vi "Lab Panel V5.22.1.vi"() -> ()   [LabVIEW 2013] (continued)
            n2200 = Equal?(x=w3894, y=w3895) -> (x = y?=w3879:bool)
            n2201 = stacked-sequence {
              tunnel: w3893 -> [w3903 _ _ _ _ _ _ _ _ _]
              tunnel: w3892 -> [_ w3979 _ _ _ _ _ _ _ _]
              tunnel: w3891 -> [_ _ w4059 _ _ _ _ _ _ _]
              tunnel: w3890 -> [_ _ _ w4139 _ _ _ _ _ _]
              tunnel: w3889 -> [_ _ _ _ w4219 _ _ _ _ _]
              tunnel: w3888 -> [_ _ _ _ _ w4299 _ _ _ _]
              tunnel: w3887 -> [_ _ _ _ _ _ w4379 _ _ _]
              tunnel: w3886 -> [_ _ _ _ _ _ _ w4459 _ _]
              tunnel: w3885 -> [_ _ _ _ _ _ _ _ w4539 _]
              tunnel: w3884 -> [_ _ _ _ _ _ _ _ _ w4619]
              tunnel: w3881 -> [w3902 w3983 w4063 w4143 w4223 w4303 w4383 w4463 w4543 w4623]
              tunnel: w3880 -> [w3901 w3982 w4062 w4142 w4222 w4302 w4382 w4462 w4542 w4622]
              tunnel: w3879 -> [w3900 w3981 w4061 w4141 w4221 w4301 w4381 w4461 w4541 w4621]
              tunnel: w3878 -> [w3899 w3980 w4060 w4140 w4220 w4300 w4380 w4460 w4540 w4620]
              frame #0 {
                n2202 = case shown="True" w3903 {
                  tunnel: w3902 -> [_ w3908]
                  tunnel: w3901 -> [_ w3907]
                  tunnel: w3900 -> [_ w3905]
                  tunnel: w3899 -> [_ w3904]
                  frame False {
                  }
                  frame True {
                    n2203 = local read "DISP LAB01-1"() -> (w3909:T4)
                    n2204 = local read "SIG LAB01-1"() -> (w3910:T2)
                    n2205 = local read "ON L01-1"() -> (w3906:cluster{"amps":dbl, "volts":dbl, "pf":dbl})
                    n2206 = Unbundle(w3910) -> ("AMPS"=w3916:dbl, "VOLTS"=w3914:dbl, "PF"=w3913:dbl, "Tmp Live"=w3912:dbl, "Tmp Neut"=w3915:dbl)
                    n2207 = Unbundle(w3909) -> ("CYCLE"=w3911:dbl)  [unwired: 2 out]
                    n2208 = stacked-sequence {
                      tunnel: w3916 -> [w3920 w3939]
                      tunnel: w3915 -> [_ w3938]
                      tunnel: w3914 -> [w3919 w3937]
                      tunnel: w3913 -> [w3918 w3936]
                      tunnel: w3912 -> [_ w3935]
                      tunnel: w3911 -> [_ w3934]
                      tunnel: w3908 -> [_ w3933]
                      tunnel: w3907 -> [w3921 _]
                      tunnel: w3906 -> [w3917 w3931]
                      tunnel: w3905 -> [_ w3932]
                      tunnel: w3904 -> [_ w3927]
                      frame #0 {
                        n2209 = case shown="True" w3921 {
                          tunnel: w3920 -> [_ w3926]
                          tunnel: w3919 -> [_ w3925]
                          tunnel: w3918 -> [_ w3924]
                          tunnel: w3917 -> [_ w3922]
                          frame False {
                          }
                          frame True {
                            n2210 = Bundle(cluster=w3922, "amps"=w3926, "volts"=w3925, "pf"=w3924) -> (w3923:cluster{"amps":dbl, "volts":dbl, "pf":dbl})
                            n2211 = local write "ON L01-1"(w3923) -> ()
                          }
                        }
                      }
                      frame #1 {
                        n2212 = Unbundle(w3931) -> ("amps"=w3930:dbl, "volts"=w3929:dbl, "pf"=w3928:dbl)
                        n2213 = case shown="True" w3932 {
                          tunnel: w3939 -> [_ w3940]
                          tunnel: w3938 -> [_ w3978]
                          tunnel: w3937 -> [_ _]
                          tunnel: w3936 -> [_ _]
                          tunnel: w3935 -> [_ w3977]
                          tunnel: w3934 -> [_ w3976]
                          tunnel: w3933 -> [_ w3944]
                          tunnel: w3930 -> [_ w3941]
                          tunnel: w3929 -> [_ w3973]
                          tunnel: w3928 -> [_ w3972]
                          tunnel: w3927 -> [_ w3942]
                          frame False {
                          }
                          frame True {
                            n2214 = local read "TDMS LAB01-1"() -> (w3975:refnum<k34>)
                            n2215 = Build Array(w3973) -> (w3969:dbl[])
                            n2216 = Build Array(w3972) -> (w3968:dbl[])
                            n2217 = Build Array(w3977) -> (w3967:dbl[])
                            n2218 = Build Array(w3978) -> (w3966:dbl[])
                            n2219 = Build Array(w3941) -> (w3971:dbl[])
                            n2220 = Build Array(w3940) -> (w3970:dbl[])
                            n2221 = Build Array(w3976) -> (w3965:dbl[])
                            n2222 = Build Array("AMPS ON", "AMPS OFF", "VOLTS", "PF", "TEMP Live", "TEMP Neut", "CYCLE") -> (w3949:string[])
                            n2223 = Bundle By Name("Y"=w3971, "t0"=w3942) -> (w3964:waveform(dbl))  [unwired: 1 in]
                            n2224 = Bundle By Name("Y"=w3970, "t0"=w3942) -> (w3963:waveform(dbl))  [unwired: 1 in]
                            n2225 = Bundle By Name("Y"=w3969, "t0"=w3942) -> (w3962:waveform(dbl))  [unwired: 1 in]
                            n2226 = Bundle By Name("Y"=w3968, "t0"=w3942) -> (w3961:waveform(dbl))  [unwired: 1 in]
                            n2227 = Bundle By Name("Y"=w3967, "t0"=w3942) -> (w3960:waveform(dbl))  [unwired: 1 in]
                            n2228 = Bundle By Name("Y"=w3966, "t0"=w3942) -> (w3959:waveform(dbl))  [unwired: 1 in]
                            n2229 = Bundle By Name("Y"=w3965, "t0"=w3942) -> (w3958:waveform(dbl))  [unwired: 1 in]
                            n2230 = Build Array(w3964, w3963, w3962, w3961, w3960, w3959, w3958) -> (w3957:waveform(dbl)[])
                            n2231 = TDMS Write(0:w3975, 5:"TEST VALUES", 7:w3949, 9:w3957) -> (4:w3948:refnum<k34>, 6:w3947:string, 15:w3946:errorcluster)  [unwired: 2 in, 1 out]
                            n2232 = TDMS Write(0:w3948, 5:w3947, 7:"TIME", 9:w3944, 11:w3946) -> (15:w3943:errorcluster)  [unwired: 1 in, 3 out]
                            n2233 = local write "data file error"(w3943) -> ()
                          }
                        }
                      }
                    }
                  }
                }
              }
              frame #1 {
                n2234 = case shown="True" w3979 {
                  tunnel: w3983 -> [_ w3988]
                  tunnel: w3982 -> [_ w3987]
                  tunnel: w3981 -> [_ w3985]
                  tunnel: w3980 -> [_ w3984]
                  frame False {
                  }
                  frame True {
                    n2235 = local read "DISP LAB01-2"() -> (w3989:T4)
                    n2236 = local read "SIG LAB01-2"() -> (w3990:T2)
                    n2237 = local read "ON L01-2"() -> (w3986:cluster{"amps":dbl, "volts":dbl, "pf":dbl})
                    n2238 = Unbundle(w3990) -> ("AMPS"=w3996:dbl, "VOLTS"=w3994:dbl, "PF"=w3993:dbl, "Tmp Live"=w3992:dbl, "Tmp Neut"=w3995:dbl)
                    n2239 = Unbundle(w3989) -> ("CYCLE"=w3991:dbl)  [unwired: 2 out]
                    n2240 = stacked-sequence {
                      tunnel: w3996 -> [w4000 w4019]
                      tunnel: w3995 -> [_ w4018]
                      tunnel: w3994 -> [w3999 w4017]
                      tunnel: w3993 -> [w3998 w4016]
                      tunnel: w3992 -> [_ w4015]
                      tunnel: w3991 -> [_ w4014]
                      tunnel: w3988 -> [_ w4013]
                      tunnel: w3987 -> [w4001 _]
                      tunnel: w3986 -> [w3997 w4011]
                      tunnel: w3985 -> [_ w4012]
                      tunnel: w3984 -> [_ w4007]
                      frame #0 {
                        n2241 = case shown="True" w4001 {
                          tunnel: w4000 -> [_ w4006]
                          tunnel: w3999 -> [_ w4005]
                          tunnel: w3998 -> [_ w4004]
                          tunnel: w3997 -> [_ w4002]
                          frame False {
                          }
                          frame True {
                            n2242 = Bundle(cluster=w4002, "amps"=w4006, "volts"=w4005, "pf"=w4004) -> (w4003:cluster{"amps":dbl, "volts":dbl, "pf":dbl})
                            n2243 = local write "ON L01-2"(w4003) -> ()
                          }
                        }
                      }
                      frame #1 {
                        n2244 = Unbundle(w4011) -> ("amps"=w4010:dbl, "volts"=w4009:dbl, "pf"=w4008:dbl)
                        n2245 = case shown="True" w4012 {
                          tunnel: w4019 -> [_ w4051]
                          tunnel: w4018 -> [_ w4058]
                          tunnel: w4017 -> [_ _]
                          tunnel: w4016 -> [_ _]
                          tunnel: w4015 -> [_ w4057]
                          tunnel: w4014 -> [_ w4056]
                          tunnel: w4013 -> [_ w4021]
                          tunnel: w4010 -> [_ w4053]
                          tunnel: w4009 -> [_ w4052]
                          tunnel: w4008 -> [_ w4050]
                          tunnel: w4007 -> [_ w4042]
                          frame False {
                          }
                          frame True {
                            n2246 = local read "TDMS LAB01-2"() -> (w4055:refnum<k34>)
                            n2247 = Build Array(w4052) -> (w4047:dbl[])
                            n2248 = Build Array(w4050) -> (w4046:dbl[])
                            n2249 = Build Array(w4057) -> (w4045:dbl[])
                            n2250 = Build Array(w4058) -> (w4044:dbl[])
                            n2251 = Build Array(w4053) -> (w4049:dbl[])
                            n2252 = Build Array(w4051) -> (w4048:dbl[])
                            n2253 = Build Array(w4056) -> (w4043:dbl[])
                            n2254 = Build Array("AMPS ON", "AMPS OFF", "VOLTS", "PF", "TEMP Live", "TEMP Neut", "CYCLE") -> (w4026:string[])
                            n2255 = Bundle By Name("Y"=w4049, "t0"=w4042) -> (w4041:waveform(dbl))  [unwired: 1 in]
                            n2256 = Bundle By Name("Y"=w4048, "t0"=w4042) -> (w4040:waveform(dbl))  [unwired: 1 in]
                            n2257 = Bundle By Name("Y"=w4047, "t0"=w4042) -> (w4039:waveform(dbl))  [unwired: 1 in]
                            n2258 = Bundle By Name("Y"=w4046, "t0"=w4042) -> (w4038:waveform(dbl))  [unwired: 1 in]
                            n2259 = Bundle By Name("Y"=w4045, "t0"=w4042) -> (w4037:waveform(dbl))  [unwired: 1 in]
                            n2260 = Bundle By Name("Y"=w4044, "t0"=w4042) -> (w4036:waveform(dbl))  [unwired: 1 in]
                            n2261 = Bundle By Name("Y"=w4043, "t0"=w4042) -> (w4035:waveform(dbl))  [unwired: 1 in]
                            n2262 = Build Array(w4041, w4040, w4039, w4038, w4037, w4036, w4035) -> (w4034:waveform(dbl)[])
                            n2263 = TDMS Write(0:w4055, 5:"TEST VALUES", 7:w4026, 9:w4034) -> (4:w4025:refnum<k34>, 6:w4024:string, 15:w4023:errorcluster)  [unwired: 2 in, 1 out]
                            n2264 = TDMS Write(0:w4025, 5:w4024, 7:"TIME", 9:w4021, 11:w4023) -> (15:w4020:errorcluster)  [unwired: 1 in, 3 out]
                            n2265 = local write "data file error"(w4020) -> ()
                          }
                        }
                      }
                    }
                  }
                }
              }
              frame #2 {
                n2266 = case shown="True" w4059 {
                  tunnel: w4063 -> [_ w4068]
                  tunnel: w4062 -> [_ w4067]
                  tunnel: w4061 -> [_ w4065]
                  tunnel: w4060 -> [_ w4064]
                  frame False {
                  }
                  frame True {
                    n2267 = local read "DISP LAB02-1"() -> (w4069:T4)
                    n2268 = local read "SIG LAB02-1"() -> (w4070:T2)
                    n2269 = local read "ON L02-1"() -> (w4066:cluster{"amps":dbl, "volts":dbl, "pf":dbl})
                    n2270 = Unbundle(w4070) -> ("AMPS"=w4076:dbl, "VOLTS"=w4074:dbl, "PF"=w4073:dbl, "Tmp Live"=w4072:dbl, "Tmp Neut"=w4075:dbl)
                    n2271 = Unbundle(w4069) -> ("CYCLE"=w4071:dbl)  [unwired: 2 out]
                    n2272 = stacked-sequence {
                      tunnel: w4076 -> [w4080 w4099]
                      tunnel: w4075 -> [_ w4098]
                      tunnel: w4074 -> [w4079 w4097]
                      tunnel: w4073 -> [w4078 w4096]
                      tunnel: w4072 -> [_ w4095]
                      tunnel: w4071 -> [_ w4094]
                      tunnel: w4068 -> [_ w4093]
                      tunnel: w4067 -> [w4081 _]
                      tunnel: w4066 -> [w4077 w4091]
                      tunnel: w4065 -> [_ w4092]
                      tunnel: w4064 -> [_ w4087]
                      frame #0 {
                        n2273 = case shown="True" w4081 {
                          tunnel: w4080 -> [_ w4086]
                          tunnel: w4079 -> [_ w4085]
                          tunnel: w4078 -> [_ w4084]
                          tunnel: w4077 -> [_ w4082]
                          frame False {
                          }
                          frame True {
                            n2274 = Bundle(cluster=w4082, "amps"=w4086, "volts"=w4085, "pf"=w4084) -> (w4083:cluster{"amps":dbl, "volts":dbl, "pf":dbl})
                            n2275 = local write "ON L02-1"(w4083) -> ()
                          }
                        }
                      }
                      frame #1 {
                        n2276 = Unbundle(w4091) -> ("amps"=w4090:dbl, "volts"=w4089:dbl, "pf"=w4088:dbl)
                        n2277 = case shown="True" w4092 {
                          tunnel: w4099 -> [_ w4131]
                          tunnel: w4098 -> [_ w4138]
                          tunnel: w4097 -> [_ _]
                          tunnel: w4096 -> [_ _]
                          tunnel: w4095 -> [_ w4137]
                          tunnel: w4094 -> [_ w4136]
                          tunnel: w4093 -> [_ w4101]
                          tunnel: w4090 -> [_ w4133]
                          tunnel: w4089 -> [_ w4132]
                          tunnel: w4088 -> [_ w4130]
                          tunnel: w4087 -> [_ w4122]
                          frame False {
                          }
                          frame True {
                            n2278 = local read "TDMS LAB02-1"() -> (w4135:refnum<k34>)
                            n2279 = Build Array(w4132) -> (w4127:dbl[])
                            n2280 = Build Array(w4130) -> (w4126:dbl[])
                            n2281 = Build Array(w4137) -> (w4125:dbl[])
                            n2282 = Build Array(w4138) -> (w4124:dbl[])
                            n2283 = Build Array(w4133) -> (w4129:dbl[])
                            n2284 = Build Array(w4131) -> (w4128:dbl[])
                            n2285 = Build Array(w4136) -> (w4123:dbl[])
                            n2286 = Build Array("AMPS ON", "AMPS OFF", "VOLTS", "PF", "TEMP Live", "TEMP Neut", "CYCLE") -> (w4106:string[])
                            n2287 = Bundle By Name("Y"=w4129, "t0"=w4122) -> (w4121:waveform(dbl))  [unwired: 1 in]
                            n2288 = Bundle By Name("Y"=w4128, "t0"=w4122) -> (w4120:waveform(dbl))  [unwired: 1 in]
                            n2289 = Bundle By Name("Y"=w4127, "t0"=w4122) -> (w4119:waveform(dbl))  [unwired: 1 in]
                            n2290 = Bundle By Name("Y"=w4126, "t0"=w4122) -> (w4118:waveform(dbl))  [unwired: 1 in]
                            n2291 = Bundle By Name("Y"=w4125, "t0"=w4122) -> (w4117:waveform(dbl))  [unwired: 1 in]
                            n2292 = Bundle By Name("Y"=w4124, "t0"=w4122) -> (w4116:waveform(dbl))  [unwired: 1 in]
                            n2293 = Bundle By Name("Y"=w4123, "t0"=w4122) -> (w4115:waveform(dbl))  [unwired: 1 in]
                            n2294 = Build Array(w4121, w4120, w4119, w4118, w4117, w4116, w4115) -> (w4114:waveform(dbl)[])
                            n2295 = TDMS Write(0:w4135, 5:"TEST VALUES", 7:w4106, 9:w4114) -> (4:w4105:refnum<k34>, 6:w4104:string, 15:w4103:errorcluster)  [unwired: 2 in, 1 out]
                            n2296 = TDMS Write(0:w4105, 5:w4104, 7:"TIME", 9:w4101, 11:w4103) -> (15:w4100:errorcluster)  [unwired: 1 in, 3 out]
                            n2297 = local write "data file error"(w4100) -> ()
                          }
                        }
                      }
                    }
                  }
                }
              }
              frame #3 {
                n2298 = case shown="True" w4139 {
                  tunnel: w4143 -> [_ w4148]
                  tunnel: w4142 -> [_ w4147]
                  tunnel: w4141 -> [_ w4145]
                  tunnel: w4140 -> [_ w4144]
                  frame False {
                  }
                  frame True {
                    n2299 = local read "DISP LAB02-2"() -> (w4149:T4)
                    n2300 = local read "SIG LAB02-2"() -> (w4150:T2)
                    n2301 = local read "ON L02-2"() -> (w4146:cluster{"amps":dbl, "volts":dbl, "pf":dbl})
                    n2302 = Unbundle(w4150) -> ("AMPS"=w4156:dbl, "VOLTS"=w4154:dbl, "PF"=w4153:dbl, "Tmp Live"=w4152:dbl, "Tmp Neut"=w4155:dbl)
                    n2303 = Unbundle(w4149) -> ("CYCLE"=w4151:dbl)  [unwired: 2 out]
                    n2304 = stacked-sequence {
                      tunnel: w4156 -> [w4160 w4179]
                      tunnel: w4155 -> [_ w4178]
                      tunnel: w4154 -> [w4159 w4177]
                      tunnel: w4153 -> [w4158 w4176]
                      tunnel: w4152 -> [_ w4175]
                      tunnel: w4151 -> [_ w4174]
                      tunnel: w4148 -> [_ w4173]
                      tunnel: w4147 -> [w4161 _]
                      tunnel: w4146 -> [w4157 w4171]
                      tunnel: w4145 -> [_ w4172]
                      tunnel: w4144 -> [_ w4167]
                      frame #0 {
                        n2305 = case shown="True" w4161 {
                          tunnel: w4160 -> [_ w4166]
                          tunnel: w4159 -> [_ w4165]
                          tunnel: w4158 -> [_ w4164]
                          tunnel: w4157 -> [_ w4162]
                          frame False {
                          }
                          frame True {
                            n2306 = Bundle(cluster=w4162, "amps"=w4166, "volts"=w4165, "pf"=w4164) -> (w4163:cluster{"amps":dbl, "volts":dbl, "pf":dbl})
                            n2307 = local write "ON L02-2"(w4163) -> ()
                          }
                        }
                      }
                      frame #1 {
                        n2308 = Unbundle(w4171) -> ("amps"=w4170:dbl, "volts"=w4169:dbl, "pf"=w4168:dbl)
                        n2309 = case shown="True" w4172 {
                          tunnel: w4179 -> [_ w4211]
                          tunnel: w4178 -> [_ w4218]
                          tunnel: w4177 -> [_ _]
                          tunnel: w4176 -> [_ _]
                          tunnel: w4175 -> [_ w4217]
                          tunnel: w4174 -> [_ w4216]
                          tunnel: w4173 -> [_ w4181]
                          tunnel: w4170 -> [_ w4213]
                          tunnel: w4169 -> [_ w4212]
                          tunnel: w4168 -> [_ w4210]
                          tunnel: w4167 -> [_ w4202]
                          frame False {
                          }
                          frame True {
                            n2310 = local read "TDMS LAB02-2"() -> (w4215:refnum<k34>)
                            n2311 = Build Array(w4212) -> (w4207:dbl[])
                            n2312 = Build Array(w4210) -> (w4206:dbl[])
                            n2313 = Build Array(w4217) -> (w4205:dbl[])
                            n2314 = Build Array(w4218) -> (w4204:dbl[])
                            n2315 = Build Array(w4213) -> (w4209:dbl[])
                            n2316 = Build Array(w4211) -> (w4208:dbl[])
                            n2317 = Build Array(w4216) -> (w4203:dbl[])
                            n2318 = Build Array("AMPS ON", "AMPS OFF", "VOLTS", "PF", "TEMP Live", "TEMP Neut", "CYCLE") -> (w4186:string[])
                            n2319 = Bundle By Name("Y"=w4209, "t0"=w4202) -> (w4201:waveform(dbl))  [unwired: 1 in]
                            n2320 = Bundle By Name("Y"=w4208, "t0"=w4202) -> (w4200:waveform(dbl))  [unwired: 1 in]
                            n2321 = Bundle By Name("Y"=w4207, "t0"=w4202) -> (w4199:waveform(dbl))  [unwired: 1 in]
                            n2322 = Bundle By Name("Y"=w4206, "t0"=w4202) -> (w4198:waveform(dbl))  [unwired: 1 in]
                            n2323 = Bundle By Name("Y"=w4205, "t0"=w4202) -> (w4197:waveform(dbl))  [unwired: 1 in]
                            n2324 = Bundle By Name("Y"=w4204, "t0"=w4202) -> (w4196:waveform(dbl))  [unwired: 1 in]
                            n2325 = Bundle By Name("Y"=w4203, "t0"=w4202) -> (w4195:waveform(dbl))  [unwired: 1 in]
                            n2326 = Build Array(w4201, w4200, w4199, w4198, w4197, w4196, w4195) -> (w4194:waveform(dbl)[])
                            n2327 = TDMS Write(0:w4215, 5:"TEST VALUES", 7:w4186, 9:w4194) -> (4:w4185:refnum<k34>, 6:w4184:string, 15:w4183:errorcluster)  [unwired: 2 in, 1 out]
                            n2328 = TDMS Write(0:w4185, 5:w4184, 7:"TIME", 9:w4181, 11:w4183) -> (15:w4180:errorcluster)  [unwired: 1 in, 3 out]
                            n2329 = local write "data file error"(w4180) -> ()
                          }
                        }
                      }
                    }
                  }
                }
              }
              frame #4 {
                n2330 = case shown="True" w4219 {
                  tunnel: w4223 -> [_ w4228]
                  tunnel: w4222 -> [_ w4227]
                  tunnel: w4221 -> [_ w4225]
                  tunnel: w4220 -> [_ w4224]
                  frame False {
                  }
                  frame True {
                    n2331 = local read "DISP LAB03-1"() -> (w4229:T4)
                    n2332 = local read "SIG LAB03-1"() -> (w4230:T2)
                    n2333 = local read "ON L03-1"() -> (w4226:cluster{"amps":dbl, "volts":dbl, "pf":dbl})
                    n2334 = Unbundle(w4230) -> ("AMPS"=w4236:dbl, "VOLTS"=w4234:dbl, "PF"=w4233:dbl, "Tmp Live"=w4232:dbl, "Tmp Neut"=w4235:dbl)
                    n2335 = Unbundle(w4229) -> ("CYCLE"=w4231:dbl)  [unwired: 2 out]
                    n2336 = stacked-sequence {
                      tunnel: w4236 -> [w4240 w4259]
                      tunnel: w4235 -> [_ w4258]
                      tunnel: w4234 -> [w4239 w4257]
                      tunnel: w4233 -> [w4238 w4256]
                      tunnel: w4232 -> [_ w4255]
                      tunnel: w4231 -> [_ w4254]
                      tunnel: w4228 -> [_ w4253]
                      tunnel: w4227 -> [w4241 _]
                      tunnel: w4226 -> [w4237 w4251]
                      tunnel: w4225 -> [_ w4252]
                      tunnel: w4224 -> [_ w4247]
                      frame #0 {
                        n2337 = case shown="True" w4241 {
                          tunnel: w4240 -> [_ w4246]
                          tunnel: w4239 -> [_ w4245]
                          tunnel: w4238 -> [_ w4244]
                          tunnel: w4237 -> [_ w4242]
                          frame False {
                          }
                          frame True {
                            n2338 = Bundle(cluster=w4242, "amps"=w4246, "volts"=w4245, "pf"=w4244) -> (w4243:cluster{"amps":dbl, "volts":dbl, "pf":dbl})
                            n2339 = local write "ON L03-1"(w4243) -> ()
                          }
                        }
                      }
                      frame #1 {
                        n2340 = Unbundle(w4251) -> ("amps"=w4250:dbl, "volts"=w4249:dbl, "pf"=w4248:dbl)
                        n2341 = case shown="True" w4252 {
                          tunnel: w4259 -> [_ w4291]
                          tunnel: w4258 -> [_ w4298]
                          tunnel: w4257 -> [_ _]
                          tunnel: w4256 -> [_ _]
                          tunnel: w4255 -> [_ w4297]
                          tunnel: w4254 -> [_ w4296]
                          tunnel: w4253 -> [_ w4261]
                          tunnel: w4250 -> [_ w4293]
                          tunnel: w4249 -> [_ w4292]
                          tunnel: w4248 -> [_ w4290]
                          tunnel: w4247 -> [_ w4282]
                          frame False {
                          }
                          frame True {
                            n2342 = local read "TDMS LAB03-1"() -> (w4295:refnum<k34>)
                            n2343 = Build Array(w4292) -> (w4287:dbl[])
                            n2344 = Build Array(w4290) -> (w4286:dbl[])
                            n2345 = Build Array(w4297) -> (w4285:dbl[])
                            n2346 = Build Array(w4298) -> (w4284:dbl[])
                            n2347 = Build Array(w4293) -> (w4289:dbl[])
                            n2348 = Build Array(w4291) -> (w4288:dbl[])
                            n2349 = Build Array(w4296) -> (w4283:dbl[])
                            n2350 = Build Array("AMPS ON", "AMPS OFF", "VOLTS", "PF", "TEMP Live", "TEMP Neut", "CYCLE") -> (w4266:string[])
                            n2351 = Bundle By Name("Y"=w4289, "t0"=w4282) -> (w4281:waveform(dbl))  [unwired: 1 in]
                            n2352 = Bundle By Name("Y"=w4288, "t0"=w4282) -> (w4280:waveform(dbl))  [unwired: 1 in]
                            n2353 = Bundle By Name("Y"=w4287, "t0"=w4282) -> (w4279:waveform(dbl))  [unwired: 1 in]
                            n2354 = Bundle By Name("Y"=w4286, "t0"=w4282) -> (w4278:waveform(dbl))  [unwired: 1 in]
                            n2355 = Bundle By Name("Y"=w4285, "t0"=w4282) -> (w4277:waveform(dbl))  [unwired: 1 in]
                            n2356 = Bundle By Name("Y"=w4284, "t0"=w4282) -> (w4276:waveform(dbl))  [unwired: 1 in]
                            n2357 = Bundle By Name("Y"=w4283, "t0"=w4282) -> (w4275:waveform(dbl))  [unwired: 1 in]
                            n2358 = Build Array(w4281, w4280, w4279, w4278, w4277, w4276, w4275) -> (w4274:waveform(dbl)[])
                            n2359 = TDMS Write(0:w4295, 5:"TEST VALUES", 7:w4266, 9:w4274) -> (4:w4265:refnum<k34>, 6:w4264:string, 15:w4263:errorcluster)  [unwired: 2 in, 1 out]
                            n2360 = TDMS Write(0:w4265, 5:w4264, 7:"TIME", 9:w4261, 11:w4263) -> (15:w4260:errorcluster)  [unwired: 1 in, 3 out]
                            n2361 = local write "data file error"(w4260) -> ()
                          }
                        }
                      }
                    }
                  }
                }
              }
              frame #5 {
                n2362 = case shown="True" w4299 {
                  tunnel: w4303 -> [_ w4308]
                  tunnel: w4302 -> [_ w4307]
                  tunnel: w4301 -> [_ w4305]
                  tunnel: w4300 -> [_ w4304]
                  frame False {
                  }
                  frame True {
                    n2363 = local read "DISP LAB03-2"() -> (w4309:T4)
                    n2364 = local read "SIG LAB03-2"() -> (w4310:T2)
                    n2365 = local read "ON L03-2"() -> (w4306:cluster{"amps":dbl, "volts":dbl, "pf":dbl})
                    n2366 = Unbundle(w4310) -> ("AMPS"=w4316:dbl, "VOLTS"=w4314:dbl, "PF"=w4313:dbl, "Tmp Live"=w4312:dbl, "Tmp Neut"=w4315:dbl)
                    n2367 = Unbundle(w4309) -> ("CYCLE"=w4311:dbl)  [unwired: 2 out]
                    n2368 = stacked-sequence {
                      tunnel: w4316 -> [w4320 w4339]
                      tunnel: w4315 -> [_ w4338]
                      tunnel: w4314 -> [w4319 w4337]
                      tunnel: w4313 -> [w4318 w4336]
                      tunnel: w4312 -> [_ w4335]
                      tunnel: w4311 -> [_ w4334]
                      tunnel: w4308 -> [_ w4333]
                      tunnel: w4307 -> [w4321 _]
                      tunnel: w4306 -> [w4317 w4331]
                      tunnel: w4305 -> [_ w4332]
                      tunnel: w4304 -> [_ w4327]
                      frame #0 {
                        n2369 = case shown="True" w4321 {
                          tunnel: w4320 -> [_ w4326]
                          tunnel: w4319 -> [_ w4325]
                          tunnel: w4318 -> [_ w4324]
                          tunnel: w4317 -> [_ w4322]
                          frame False {
                          }
                          frame True {
                            n2370 = Bundle(cluster=w4322, "amps"=w4326, "volts"=w4325, "pf"=w4324) -> (w4323:cluster{"amps":dbl, "volts":dbl, "pf":dbl})
                            n2371 = local write "ON L03-2"(w4323) -> ()
                          }
                        }
                      }
                      frame #1 {
                        n2372 = Unbundle(w4331) -> ("amps"=w4330:dbl, "volts"=w4329:dbl, "pf"=w4328:dbl)
                        n2373 = case shown="True" w4332 {
                          tunnel: w4339 -> [_ w4371]
                          tunnel: w4338 -> [_ w4378]
                          tunnel: w4337 -> [_ _]
                          tunnel: w4336 -> [_ _]
                          tunnel: w4335 -> [_ w4377]
                          tunnel: w4334 -> [_ w4376]
                          tunnel: w4333 -> [_ w4341]
                          tunnel: w4330 -> [_ w4373]
                          tunnel: w4329 -> [_ w4372]
                          tunnel: w4328 -> [_ w4370]
                          tunnel: w4327 -> [_ w4362]
                          frame False {
                          }
                          frame True {
                            n2374 = local read "TDMS LAB03-2"() -> (w4375:refnum<k34>)
                            n2375 = Build Array(w4372) -> (w4367:dbl[])
                            n2376 = Build Array(w4370) -> (w4366:dbl[])
                            n2377 = Build Array(w4377) -> (w4365:dbl[])
                            n2378 = Build Array(w4378) -> (w4364:dbl[])
                            n2379 = Build Array(w4373) -> (w4369:dbl[])
                            n2380 = Build Array(w4371) -> (w4368:dbl[])
                            n2381 = Build Array(w4376) -> (w4363:dbl[])
                            n2382 = Build Array("AMPS ON", "AMPS OFF", "VOLTS", "PF", "TEMP Live", "TEMP Neut", "CYCLE") -> (w4346:string[])
                            n2383 = Bundle By Name("Y"=w4369, "t0"=w4362) -> (w4361:waveform(dbl))  [unwired: 1 in]
                            n2384 = Bundle By Name("Y"=w4368, "t0"=w4362) -> (w4360:waveform(dbl))  [unwired: 1 in]
                            n2385 = Bundle By Name("Y"=w4367, "t0"=w4362) -> (w4359:waveform(dbl))  [unwired: 1 in]
                            n2386 = Bundle By Name("Y"=w4366, "t0"=w4362) -> (w4358:waveform(dbl))  [unwired: 1 in]
                            n2387 = Bundle By Name("Y"=w4365, "t0"=w4362) -> (w4357:waveform(dbl))  [unwired: 1 in]
                            n2388 = Bundle By Name("Y"=w4364, "t0"=w4362) -> (w4356:waveform(dbl))  [unwired: 1 in]
                            n2389 = Bundle By Name("Y"=w4363, "t0"=w4362) -> (w4355:waveform(dbl))  [unwired: 1 in]
                            n2390 = Build Array(w4361, w4360, w4359, w4358, w4357, w4356, w4355) -> (w4354:waveform(dbl)[])
                            n2391 = TDMS Write(0:w4375, 5:"TEST VALUES", 7:w4346, 9:w4354) -> (4:w4345:refnum<k34>, 6:w4344:string, 15:w4343:errorcluster)  [unwired: 2 in, 1 out]
                            n2392 = TDMS Write(0:w4345, 5:w4344, 7:"TIME", 9:w4341, 11:w4343) -> (15:w4340:errorcluster)  [unwired: 1 in, 3 out]
                            n2393 = local write "data file error"(w4340) -> ()
                          }
                        }
                      }
                    }
                  }
                }
              }
              frame #6 {
                n2394 = case shown="True" w4379 {
                  tunnel: w4383 -> [_ w4388]
                  tunnel: w4382 -> [_ w4387]
                  tunnel: w4381 -> [_ w4385]
                  tunnel: w4380 -> [_ w4384]
                  frame False {
                  }
                  frame True {
                    n2395 = local read "DISP LAB04-1"() -> (w4389:T4)
                    n2396 = local read "SIG LAB04-1"() -> (w4390:T2)
                    n2397 = local read "ON L04-1"() -> (w4386:cluster{"amps":dbl, "volts":dbl, "pf":dbl})
                    n2398 = Unbundle(w4390) -> ("AMPS"=w4396:dbl, "VOLTS"=w4394:dbl, "PF"=w4393:dbl, "Tmp Live"=w4392:dbl, "Tmp Neut"=w4395:dbl)
                    n2399 = Unbundle(w4389) -> ("CYCLE"=w4391:dbl)  [unwired: 2 out]
                    n2400 = stacked-sequence {
                      tunnel: w4396 -> [w4400 w4419]
                      tunnel: w4395 -> [_ w4418]
                      tunnel: w4394 -> [w4399 w4417]
                      tunnel: w4393 -> [w4398 w4416]
                      tunnel: w4392 -> [_ w4415]
                      tunnel: w4391 -> [_ w4414]
                      tunnel: w4388 -> [_ w4413]
                      tunnel: w4387 -> [w4401 _]
                      tunnel: w4386 -> [w4397 w4411]
                      tunnel: w4385 -> [_ w4412]
                      tunnel: w4384 -> [_ w4407]
                      frame #0 {
                        n2401 = case shown="True" w4401 {
                          tunnel: w4400 -> [_ w4406]
                          tunnel: w4399 -> [_ w4405]
                          tunnel: w4398 -> [_ w4404]
                          tunnel: w4397 -> [_ w4402]
                          frame False {
                          }
                          frame True {
                            n2402 = Bundle(cluster=w4402, "amps"=w4406, "volts"=w4405, "pf"=w4404) -> (w4403:cluster{"amps":dbl, "volts":dbl, "pf":dbl})
                            n2403 = local write "ON L04-1"(w4403) -> ()
                          }
                        }
                      }
                      frame #1 {
                        n2404 = Unbundle(w4411) -> ("amps"=w4410:dbl, "volts"=w4409:dbl, "pf"=w4408:dbl)
                        n2405 = case shown="True" w4412 {
                          tunnel: w4419 -> [_ w4451]
                          tunnel: w4418 -> [_ w4458]
                          tunnel: w4417 -> [_ _]
                          tunnel: w4416 -> [_ _]
                          tunnel: w4415 -> [_ w4457]
                          tunnel: w4414 -> [_ w4456]
                          tunnel: w4413 -> [_ w4421]
                          tunnel: w4410 -> [_ w4453]
                          tunnel: w4409 -> [_ w4452]
                          tunnel: w4408 -> [_ w4450]
                          tunnel: w4407 -> [_ w4442]
                          frame False {
                          }
                          frame True {
                            n2406 = local read "TDMS LAB04-1"() -> (w4455:refnum<k34>)
                            n2407 = Build Array(w4452) -> (w4447:dbl[])
                            n2408 = Build Array(w4450) -> (w4446:dbl[])
                            n2409 = Build Array(w4457) -> (w4445:dbl[])
                            n2410 = Build Array(w4458) -> (w4444:dbl[])
                            n2411 = Build Array(w4453) -> (w4449:dbl[])
                            n2412 = Build Array(w4451) -> (w4448:dbl[])
                            n2413 = Build Array(w4456) -> (w4443:dbl[])
                            n2414 = Build Array("AMPS ON", "AMPS OFF", "VOLTS", "PF", "TEMP Live", "TEMP Neut", "CYCLE") -> (w4426:string[])
                            n2415 = Bundle By Name("Y"=w4449, "t0"=w4442) -> (w4441:waveform(dbl))  [unwired: 1 in]
                            n2416 = Bundle By Name("Y"=w4448, "t0"=w4442) -> (w4440:waveform(dbl))  [unwired: 1 in]
                            n2417 = Bundle By Name("Y"=w4447, "t0"=w4442) -> (w4439:waveform(dbl))  [unwired: 1 in]
                            n2418 = Bundle By Name("Y"=w4446, "t0"=w4442) -> (w4438:waveform(dbl))  [unwired: 1 in]
                            n2419 = Bundle By Name("Y"=w4445, "t0"=w4442) -> (w4437:waveform(dbl))  [unwired: 1 in]
                            n2420 = Bundle By Name("Y"=w4444, "t0"=w4442) -> (w4436:waveform(dbl))  [unwired: 1 in]
                            n2421 = Bundle By Name("Y"=w4443, "t0"=w4442) -> (w4435:waveform(dbl))  [unwired: 1 in]
                            n2422 = Build Array(w4441, w4440, w4439, w4438, w4437, w4436, w4435) -> (w4434:waveform(dbl)[])
                            n2423 = TDMS Write(0:w4455, 5:"TEST VALUES", 7:w4426, 9:w4434) -> (4:w4425:refnum<k34>, 6:w4424:string, 15:w4423:errorcluster)  [unwired: 2 in, 1 out]
                            n2424 = TDMS Write(0:w4425, 5:w4424, 7:"TIME", 9:w4421, 11:w4423) -> (15:w4420:errorcluster)  [unwired: 1 in, 3 out]
                            n2425 = local write "data file error"(w4420) -> ()
                          }
                        }
                      }
                    }
                  }
                }
              }
              frame #7 {
                n2426 = case shown="True" w4459 {
                  tunnel: w4463 -> [_ w4468]
                  tunnel: w4462 -> [_ w4467]
                  tunnel: w4461 -> [_ w4465]
                  tunnel: w4460 -> [_ w4464]
                  frame False {
                  }
                  frame True {
                    n2427 = local read "DISP LAB04-2"() -> (w4469:T4)
                    n2428 = local read "SIG LAB04-2"() -> (w4470:T2)
                    n2429 = local read "ON L04-2"() -> (w4466:cluster{"amps":dbl, "volts":dbl, "pf":dbl})
                    n2430 = Unbundle(w4470) -> ("AMPS"=w4476:dbl, "VOLTS"=w4474:dbl, "PF"=w4473:dbl, "Tmp Live"=w4472:dbl, "Tmp Neut"=w4475:dbl)
                    n2431 = Unbundle(w4469) -> ("CYCLE"=w4471:dbl)  [unwired: 2 out]
                    n2432 = stacked-sequence {
                      tunnel: w4476 -> [w4480 w4499]
                      tunnel: w4475 -> [_ w4498]
                      tunnel: w4474 -> [w4479 w4497]
                      tunnel: w4473 -> [w4478 w4496]
                      tunnel: w4472 -> [_ w4495]
                      tunnel: w4471 -> [_ w4494]
                      tunnel: w4468 -> [_ w4493]
                      tunnel: w4467 -> [w4481 _]
                      tunnel: w4466 -> [w4477 w4491]
                      tunnel: w4465 -> [_ w4492]
                      tunnel: w4464 -> [_ w4487]
                      frame #0 {
                        n2433 = case shown="True" w4481 {
                          tunnel: w4480 -> [_ w4486]
                          tunnel: w4479 -> [_ w4485]
                          tunnel: w4478 -> [_ w4484]
                          tunnel: w4477 -> [_ w4482]
                          frame False {
                          }
                          frame True {
                            n2434 = Bundle(cluster=w4482, "amps"=w4486, "volts"=w4485, "pf"=w4484) -> (w4483:cluster{"amps":dbl, "volts":dbl, "pf":dbl})
                            n2435 = local write "ON L04-2"(w4483) -> ()
                          }
                        }
                      }
                      frame #1 {
                        n2436 = Unbundle(w4491) -> ("amps"=w4490:dbl, "volts"=w4489:dbl, "pf"=w4488:dbl)
                        n2437 = case shown="True" w4492 {
                          tunnel: w4499 -> [_ w4531]
                          tunnel: w4498 -> [_ w4538]
                          tunnel: w4497 -> [_ _]
                          tunnel: w4496 -> [_ _]
                          tunnel: w4495 -> [_ w4537]
                          tunnel: w4494 -> [_ w4536]
                          tunnel: w4493 -> [_ w4501]
                          tunnel: w4490 -> [_ w4533]
                          tunnel: w4489 -> [_ w4532]
                          tunnel: w4488 -> [_ w4530]
                          tunnel: w4487 -> [_ w4522]
                          frame False {
                          }
                          frame True {
                            n2438 = local read "TDMS LAB04-2"() -> (w4535:refnum<k34>)
                            n2439 = Build Array(w4532) -> (w4527:dbl[])
                            n2440 = Build Array(w4530) -> (w4526:dbl[])
                            n2441 = Build Array(w4537) -> (w4525:dbl[])
                            n2442 = Build Array(w4538) -> (w4524:dbl[])
                            n2443 = Build Array(w4533) -> (w4529:dbl[])
                            n2444 = Build Array(w4531) -> (w4528:dbl[])
                            n2445 = Build Array(w4536) -> (w4523:dbl[])
                            n2446 = Build Array("AMPS ON", "AMPS OFF", "VOLTS", "PF", "TEMP Live", "TEMP Neut", "CYCLE") -> (w4506:string[])
                            n2447 = Bundle By Name("Y"=w4529, "t0"=w4522) -> (w4521:waveform(dbl))  [unwired: 1 in]
                            n2448 = Bundle By Name("Y"=w4528, "t0"=w4522) -> (w4520:waveform(dbl))  [unwired: 1 in]
                            n2449 = Bundle By Name("Y"=w4527, "t0"=w4522) -> (w4519:waveform(dbl))  [unwired: 1 in]
                            n2450 = Bundle By Name("Y"=w4526, "t0"=w4522) -> (w4518:waveform(dbl))  [unwired: 1 in]
                            n2451 = Bundle By Name("Y"=w4525, "t0"=w4522) -> (w4517:waveform(dbl))  [unwired: 1 in]
                            n2452 = Bundle By Name("Y"=w4524, "t0"=w4522) -> (w4516:waveform(dbl))  [unwired: 1 in]
                            n2453 = Bundle By Name("Y"=w4523, "t0"=w4522) -> (w4515:waveform(dbl))  [unwired: 1 in]
                            n2454 = Build Array(w4521, w4520, w4519, w4518, w4517, w4516, w4515) -> (w4514:waveform(dbl)[])
                            n2455 = TDMS Write(0:w4535, 5:"TEST VALUES", 7:w4506, 9:w4514) -> (4:w4505:refnum<k34>, 6:w4504:string, 15:w4503:errorcluster)  [unwired: 2 in, 1 out]
                            n2456 = TDMS Write(0:w4505, 5:w4504, 7:"TIME", 9:w4501, 11:w4503) -> (15:w4500:errorcluster)  [unwired: 1 in, 3 out]
                            n2457 = local write "data file error"(w4500) -> ()
                          }
                        }
                      }
                    }
                  }
                }
              }
              frame #8 {
                n2458 = case shown="True" w4539 {
                  tunnel: w4543 -> [_ w4548]
                  tunnel: w4542 -> [_ w4547]
                  tunnel: w4541 -> [_ w4545]
                  tunnel: w4540 -> [_ w4544]
                  frame False {
                  }
                  frame True {
                    n2459 = local read "DISP LAB05-1"() -> (w4549:T4)
                    n2460 = local read "SIG LAB05-1"() -> (w4550:T2)
                    n2461 = local read "ON L05-1"() -> (w4546:cluster{"amps":dbl, "volts":dbl, "pf":dbl})
                    n2462 = Unbundle(w4550) -> ("AMPS"=w4556:dbl, "VOLTS"=w4554:dbl, "PF"=w4553:dbl, "Tmp Live"=w4552:dbl, "Tmp Neut"=w4555:dbl)
                    n2463 = Unbundle(w4549) -> ("CYCLE"=w4551:dbl)  [unwired: 2 out]
                    n2464 = stacked-sequence {
                      tunnel: w4556 -> [w4560 w4579]
                      tunnel: w4555 -> [_ w4578]
                      tunnel: w4554 -> [w4559 w4577]
                      tunnel: w4553 -> [w4558 w4576]
                      tunnel: w4552 -> [_ w4575]
                      tunnel: w4551 -> [_ w4574]
                      tunnel: w4548 -> [_ w4573]
                      tunnel: w4547 -> [w4561 _]
                      tunnel: w4546 -> [w4557 w4571]
                      tunnel: w4545 -> [_ w4572]
                      tunnel: w4544 -> [_ w4567]
                      frame #0 {
                        n2465 = case shown="True" w4561 {
                          tunnel: w4560 -> [_ w4566]
                          tunnel: w4559 -> [_ w4565]
                          tunnel: w4558 -> [_ w4564]
                          tunnel: w4557 -> [_ w4562]
                          frame False {
                          }
                          frame True {
                            n2466 = Bundle(cluster=w4562, "amps"=w4566, "volts"=w4565, "pf"=w4564) -> (w4563:cluster{"amps":dbl, "volts":dbl, "pf":dbl})
                            n2467 = local write "ON L05-1"(w4563) -> ()
                          }
                        }
                      }
                      frame #1 {
                        n2468 = Unbundle(w4571) -> ("amps"=w4570:dbl, "volts"=w4569:dbl, "pf"=w4568:dbl)
                        n2469 = case shown="True" w4572 {
                          tunnel: w4579 -> [_ w4611]
                          tunnel: w4578 -> [_ w4618]
                          tunnel: w4577 -> [_ _]
                          tunnel: w4576 -> [_ _]
                          tunnel: w4575 -> [_ w4617]
                          tunnel: w4574 -> [_ w4616]
                          tunnel: w4573 -> [_ w4581]
                          tunnel: w4570 -> [_ w4613]
                          tunnel: w4569 -> [_ w4612]
                          tunnel: w4568 -> [_ w4610]
                          tunnel: w4567 -> [_ w4602]
                          frame False {
                          }
                          frame True {
                            n2470 = local read "TDMS LAB05-1"() -> (w4615:refnum<k34>)
                            n2471 = Build Array(w4612) -> (w4607:dbl[])
                            n2472 = Build Array(w4610) -> (w4606:dbl[])
                            n2473 = Build Array(w4617) -> (w4605:dbl[])
                            n2474 = Build Array(w4618) -> (w4604:dbl[])
                            n2475 = Build Array(w4613) -> (w4609:dbl[])
                            n2476 = Build Array(w4611) -> (w4608:dbl[])
                            n2477 = Build Array(w4616) -> (w4603:dbl[])
                            n2478 = Build Array("AMPS ON", "AMPS OFF", "VOLTS", "PF", "TEMP Live", "TEMP Neut", "CYCLE") -> (w4586:string[])
                            n2479 = Bundle By Name("Y"=w4609, "t0"=w4602) -> (w4601:waveform(dbl))  [unwired: 1 in]
                            n2480 = Bundle By Name("Y"=w4608, "t0"=w4602) -> (w4600:waveform(dbl))  [unwired: 1 in]
                            n2481 = Bundle By Name("Y"=w4607, "t0"=w4602) -> (w4599:waveform(dbl))  [unwired: 1 in]
                            n2482 = Bundle By Name("Y"=w4606, "t0"=w4602) -> (w4598:waveform(dbl))  [unwired: 1 in]
                            n2483 = Bundle By Name("Y"=w4605, "t0"=w4602) -> (w4597:waveform(dbl))  [unwired: 1 in]
                            n2484 = Bundle By Name("Y"=w4604, "t0"=w4602) -> (w4596:waveform(dbl))  [unwired: 1 in]
                            n2485 = Bundle By Name("Y"=w4603, "t0"=w4602) -> (w4595:waveform(dbl))  [unwired: 1 in]
                            n2486 = Build Array(w4601, w4600, w4599, w4598, w4597, w4596, w4595) -> (w4594:waveform(dbl)[])
                            n2487 = TDMS Write(0:w4615, 5:"TEST VALUES", 7:w4586, 9:w4594) -> (4:w4585:refnum<k34>, 6:w4584:string, 15:w4583:errorcluster)  [unwired: 2 in, 1 out]
                            n2488 = TDMS Write(0:w4585, 5:w4584, 7:"TIME", 9:w4581, 11:w4583) -> (15:w4580:errorcluster)  [unwired: 1 in, 3 out]
                            n2489 = local write "data file error"(w4580) -> ()
                          }
                        }
                      }
                    }
                  }
                }
              }
              frame #9 {
                n2490 = case shown="True" w4619 {
                  tunnel: w4623 -> [_ w4628]
                  tunnel: w4622 -> [_ w4627]
                  tunnel: w4621 -> [_ w4625]
                  tunnel: w4620 -> [_ w4624]
                  frame False {
                  }
                  frame True {
                    n2491 = local read "DISP LAB05-2"() -> (w4629:T4)
                    n2492 = local read "SIG LAB05-2"() -> (w4630:T2)
                    n2493 = local read "ON L05-2"() -> (w4626:cluster{"amps":dbl, "volts":dbl, "pf":dbl})
                    n2494 = Unbundle(w4630) -> ("AMPS"=w4636:dbl, "VOLTS"=w4634:dbl, "PF"=w4633:dbl, "Tmp Live"=w4632:dbl, "Tmp Neut"=w4635:dbl)
                    n2495 = Unbundle(w4629) -> ("CYCLE"=w4631:dbl)  [unwired: 2 out]
                    n2496 = stacked-sequence {
                      tunnel: w4636 -> [w4640 w4659]
                      tunnel: w4635 -> [_ w4658]
                      tunnel: w4634 -> [w4639 w4657]
                      tunnel: w4633 -> [w4638 w4656]
                      tunnel: w4632 -> [_ w4655]
                      tunnel: w4631 -> [_ w4654]
                      tunnel: w4628 -> [_ w4653]
                      tunnel: w4627 -> [w4641 _]
                      tunnel: w4626 -> [w4637 w4651]
                      tunnel: w4625 -> [_ w4652]
                      tunnel: w4624 -> [_ w4647]
                      frame #0 {
                        n2497 = case shown="True" w4641 {
                          tunnel: w4640 -> [_ w4646]
                          tunnel: w4639 -> [_ w4645]
                          tunnel: w4638 -> [_ w4644]
                          tunnel: w4637 -> [_ w4642]
                          frame False {
                          }
                          frame True {
